vi "AD5781SetGlobalVariables.vi"(0 "actDACRegister":u32=1572792 caption="actRegister" format="%024b", 1 "write actDACRegister":bool, 3 "setDACRegister":u32=1572792 format="%024b", 4 "write setDACRegister":bool, 8 "DacStateCmdByHost":T1, 9 "DacState":T1, 10 "write DacStateCmdByHost":bool, 11 "write DacState":bool, 13 "dac0VRegister":u32=1572792 format="%024b", 14 "writeSpiGlobals":bool, 19 "write dac0VRegister":bool) -> ()   [LabVIEW 2014]
uses:
  Controls/DacState.ctl
  Controls/FPGA SPI_FPGA SPI State.ctl
  <vilib>/rvi/Emulation/niFpgaSctlEmulationGetInTimedLoop.vi
  Code/FPGA SPI_Globals.vi
  <vilib>/rvi/Emulation/niFpgaProcessEmulError.vi
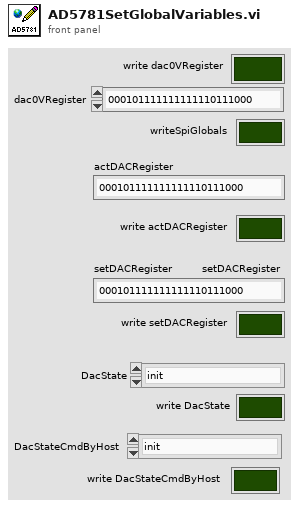
[diagram p1: front panel]
types:
  T1 = typedef "DacState.ctl" = enum16{"init", "idle", "setVolt", "error"}
  T2 = typedef "FPGA SPI_FPGA SPI State.ctl" = enum8{"Idle", "Read/Write SPI", "Configure"}
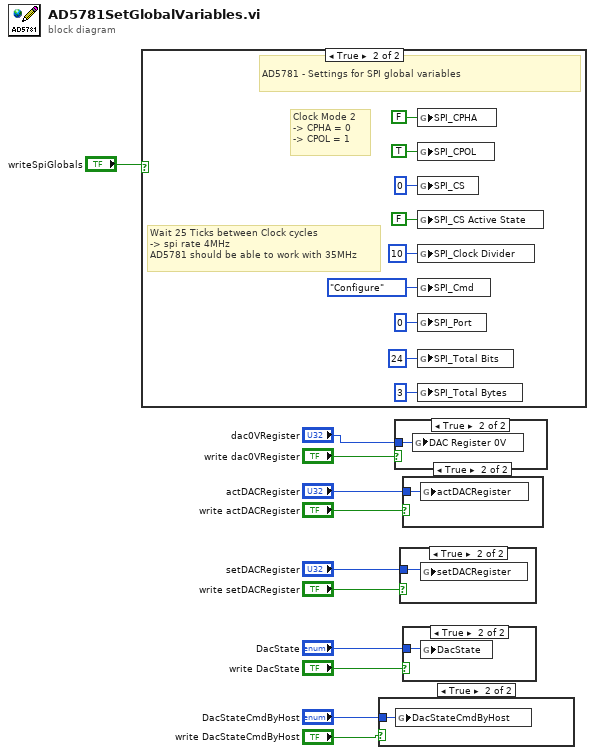
[diagram p0: block diagram]
diagram:
  n1 = case shown="True" "writeSpiGlobals" {
    frame False {
    }
    frame True {
      # "AD5781 - Settings for SPI global variables"
      # "Clock Mode 2 \n-> CPHA = 0\n-> CPOL = 1"
      # "Wait 25 Ticks between Clock cycles\n-> spi rate 4MHz\nAD5781 should be able to work with 35MHz"
      n2 = global write "FPGA SPI_Globals.vi" "SPI_CPHA"(FALSE ("SPI_CPHA")) -> ()
      n3 = global write "FPGA SPI_Globals.vi" "SPI_CPOL"(TRUE ("SPI_CPOL")) -> ()
      n4 = global write "FPGA SPI_Globals.vi" "SPI_CS"(u8 0 ("SPI_CS")) -> ()
      n5 = global write "FPGA SPI_Globals.vi" "SPI_CS Active State"(FALSE ("SPI_CS Active State")) -> ()
      n6 = global write "FPGA SPI_Globals.vi" "SPI_Clock Divider"(u32 10 ("SPI_Clock Divider")) -> ()
      n7 = global write "FPGA SPI_Globals.vi" "SPI_Cmd"(FPGA_SPI_FPGA_SPI_State."Configure" ("SPI_Cmd")) -> ()
      n8 = global write "FPGA SPI_Globals.vi" "SPI_Port"(i8 0 ("SPI_Port")) -> ()
      n9 = global write "FPGA SPI_Globals.vi" "SPI_Total Bits"(u16 24 ("SPI_Total Bits")) -> ()
      n10 = global write "FPGA SPI_Globals.vi" "SPI_Total Bytes"(u16 3 ("SPI_Total Bytes")) -> ()
    }
  }
  n11 = case shown="True" "write DacStateCmdByHost" {
    tunnel: "DacStateCmdByHost" -> [_ w21]
    frame False {
    }
    frame True {
      n12 = global write "FPGA SPI_Globals.vi" "DacStateCmdByHost"(w21) -> ()
    }
  }
  n13 = case shown="True" "write dac0VRegister" {
    tunnel: "dac0VRegister" -> [_ w22]
    frame False {
    }
    frame True {
      n14 = global write "FPGA SPI_Globals.vi" "DAC Register 0V"(w22) -> ()
    }
  }
  n15 = case shown="True" "write setDACRegister" {
    tunnel: "setDACRegister" -> [_ w23]
    frame False {
    }
    frame True {
      n16 = global write "FPGA SPI_Globals.vi" "setDACRegister"(w23) -> ()
    }
  }
  n17 = case shown="True" "write actDACRegister" {
    tunnel: "actDACRegister" -> [_ w24]
    frame False {
    }
    frame True {
      n18 = global write "FPGA SPI_Globals.vi" "actDACRegister"(w24) -> ()
    }
  }
  n19 = case shown="True" "write DacState" {
    tunnel: "DacState" -> [_ w25]
    frame False {
    }
    frame True {
      n20 = global write "FPGA SPI_Globals.vi" "DacState"(w25) -> ()
    }
  }
